vi "ATS_MS_Set_Device.vi"(8 "Update_Only":bool, 9 "Set_Manually (F)":bool, 10 "Setup_In":T1={"Record"={"Count"=1, "Presize"=512, "Length"=4096}, "Clock"={"ClckSource"=enum."Internal", "ClckRate"=12, "ClckEdge"=0, "Decimation"=0}, "Input A"={"Coupling"=enum."DC", "Range"=8, "Impedance"=enum."1M ohms", "Bandwidth"=enum."Full Bandwidth"}, "Input B"={"Coupling"=enum."DC", "Range"=8, "Impedance"=enum."1M ohms", "Bandwidth"=enum."Full Bandwidth"}, "Trigger"={"TrigOperation"=enum."X or Y", "Timeout (s)"=-1.0, "Trig. Delay"=0, "Engine X"={"Source"=enum."Chan_A", "Slope"=enum."Positive", "Level"=128}, "Engine Y"={"Source"=enum."Disable", "Slope"=enum."Positive", "Level"=128}, "ExtTrigControl"={"Coupling"=enum."AC", "Range"=enum."1 V"}}} {"Clock"."ClckEdge" items=["Rising", "Falling"]; "Clock"."ClckRate" items=["1 kS/s", "2 kS/s", "5 kS/s", "10 kS/s", "20 kS/s", "50 kS/s", "100 kS/s", "200 kS/s", "500 kS/s", "1 MS/s", "2 MS/s", "5 MS/s", "10 MS/s", "20 MS/s", "50 MS/s", "100 MS/s", "250 MS/s", "500 MS/s"]; "Input B"."Range" items=["40mV", "100mV", "200mV", "400mV", "1 V", "2 V", "4 V"]; "Trigger"."Timeout (s)" format="%.2f"; "Input A"."Range" items=["40mV", "100mV", "200mV", "400mV", "1 V", "2 V", "4 V"]}, 11 "DeviceIn":i32) -> (0 "error out":errorcluster={"status"=TRUE, "code"=60, "source"="ATS :     ApiInvalidHandle"}, 1 "Clock_Value (s)":dbl format="%.2p", 2 "Setup_Out":T1={"Record"={"Count"=1, "Presize"=512, "Length"=4096}, "Clock"={"ClckSource"=enum."Internal", "ClckRate"=12, "ClckEdge"=0, "Decimation"=0}, "Input A"={"Coupling"=enum."DC", "Range"=8, "Impedance"=enum."1M ohms", "Bandwidth"=enum."Full Bandwidth"}, "Input B"={"Coupling"=enum."DC", "Range"=8, "Impedance"=enum."1M ohms", "Bandwidth"=enum."Full Bandwidth"}, "Trigger"={"TrigOperation"=enum."X or Y", "Timeout (s)"=0.032768000000000005, "Trig. Delay"=0, "Engine X"={"Source"=enum."Chan_A", "Slope"=enum."Positive", "Level"=128}, "Engine Y"={"Source"=enum."Disable", "Slope"=enum."Positive", "Level"=128}, "ExtTrigControl"={"Coupling"=enum."AC", "Range"=enum."1 V"}}} {"Clock"."ClckEdge" items=["Rising", "Falling"]; "Clock"."ClckRate" items=["1 kS/s", "2 kS/s", "5 kS/s", "10 kS/s", "20 kS/s", "50 kS/s", "100 kS/s", "200 kS/s", "500 kS/s", "1 MS/s", "2 MS/s", "5 MS/s", "10 MS/s", "20 MS/s", "50 MS/s", "100 MS/s", "250 MS/s", "500 MS/s"]; "Input B"."Range" items=["20mv", "40mV", "50mV", "80mV", "100mV", "200mV", "400mV", "500mV", "800mV", "1 V", "2 V", "4 V", "5 V", "8 V", "10 V", "20 V"]; "Trigger"."Timeout (s)" max=0.0 format="%.2f"; "Input A"."Range" items=["20mv", "40mV", "50mV", "80mV", "100mV", "200mV", "400mV", "500mV", "800mV", "1 V", "2 V", "4 V", "5 V", "8 V", "10 V", "20 V"]}, 3 "DeviceOut":i32, 4 "TimeOut":dbl format="%.2f", 5 "#Device":i32)   [LabVIEW 2010]
doc: "_____AlazarTech, Scope_____\n\nSet ATS device with Setup_In parameters.\nIf Set_Manually is TRUE : Front panel open and the user can change setting.\nIf Set_Manually is FALSE: \n - update using input parameters.\n If UPDATE_Only is TRUE: update from previous set parameters"
uses:
  ATS_ctl/ATS_Global.ctl
  ATS_ctl/Record.ctl
  ATS_ctl/Clock.ctl
  ATS_ctl/ClockSource.ctl
  ATS_ctl/ClockRate.ctl
  ATS_ctl/ClockEdge.ctl
  ATS_ctl/InputCtrl.ctl
  ATS_ctl/Coupling.ctl
  ATS_ctl/Range.ctl
  ATS_ctl/Impedance.ctl
  ATS_ctl/Bandwidth.ctl
  ATS_ctl/Trigger.ctl
  ATS_ctl/TriggerOperation.ctl
  ATS_ctl/TriggerEngine.ctl
  ATS_ctl/ExtTrigger.ctl
  ATS_ctl/ExtTrigRange.ctl
  ATS_ctl/ATS_Spec_Selector.ctl
  ATS_ctl/ATS_Global_Ctrl.ctl
panel:
  out "Board":string
  out "Device":i32
  in  "String":string="Set parameters then push \"Continue ==>\""
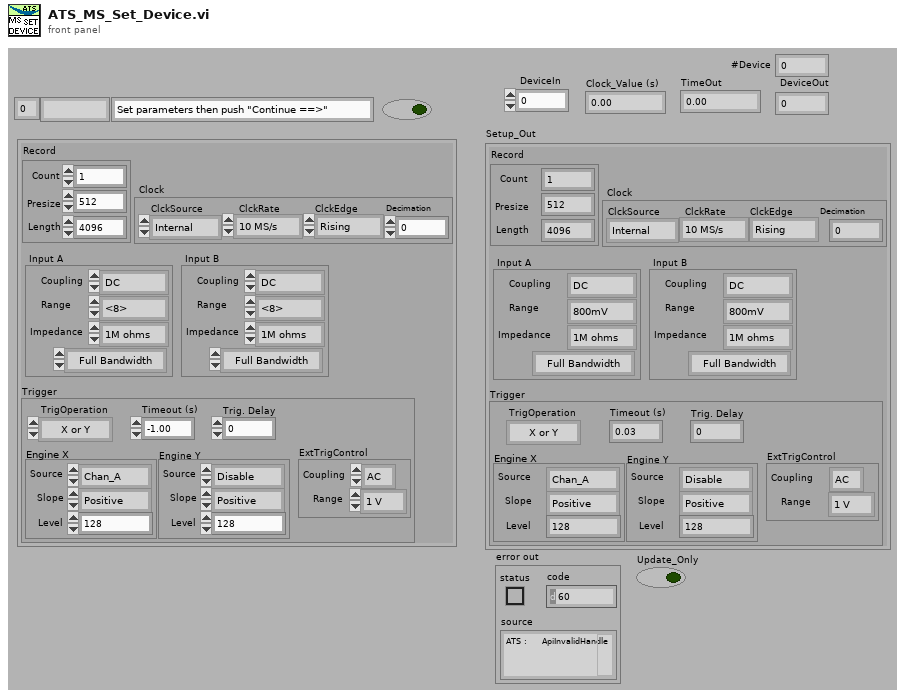
[diagram p1: front panel]
types:
  T1 = typedef "ATS_Global.ctl" = cluster{"Record":T2, "Clock":T3, "Input A":T7, "Input B":T7, "Trigger":T12}
  T2 = typedef "Record.ctl" = cluster{"Count":u32, "Presize":u32, "Length":u32}
  T3 = typedef "Clock.ctl" = cluster{"ClckSource":T4, "ClckRate":T5, "ClckEdge":T6, "Decimation":u32}
  T4 = typedef "ClockSource.ctl" = enum16{"Internal", "External", "Medium Ext.", "Slow Ext.", "Ext. AC", "Ext. DC", "Ext. (PLL)"}
  T5 = typedef "ClockRate.ctl" = u32
  T6 = typedef "ClockEdge.ctl" = u16
  T7 = typedef "InputCtrl.ctl" = cluster{"Coupling":T8, "Range":T9, "Impedance":T10, "Bandwidth":T11}
  T8 = typedef "Coupling.ctl" = enum16{"AC", "DC"}
  T9 = typedef "Range.ctl" = u32
  T10 = typedef "Impedance.ctl" = enum16{"1M ohms", "50 ohms"}
  T11 = typedef "Bandwidth.ctl" = enum16{"Full Bandwidth", "Reduce Bandwidth"}
  T12 = typedef "Trigger.ctl" = cluster{"TrigOperation":T13, "Timeout (s)":dbl, "Trig. Delay":u32, "Engine X":T14, "Engine Y":T14, "ExtTrigControl":T15}
  T13 = typedef "TriggerOperation.ctl" = enum16{"Only X", "Only Y", "X or Y", "X and Y", "X xor Y", "X and not Y", "not X and Y"}
  T14 = typedef "TriggerEngine.ctl" = cluster{"Source":enum32{"Chan_A", "Chan_B", "External", "Disable"}, "Slope":enum32{"Positive", "Negative"}, "Level":u32}
  T15 = typedef "ExtTrigger.ctl" = cluster{"Coupling":T8, "Range":T16}
  T16 = typedef "ExtTrigRange.ctl" = enum16{"1 V", "5 V", "TTL"}
  T17 = typedef "ATS_Spec_Selector.ctl" = enum16{"None", "ClckSource", "ClckEdge", "ClckRate", "InputRange", "InputCoupling", "Impedance", "Bandwidth", "AsyncDMA", "Memory", "ExtTrigCoupling", "ExtTrigRange", "AUX_IO_Trig", "AUX_IO_Slope", "Trigger_Source"}
  T18 = typedef "ATS_Global_Ctrl.ctl" = enum16{"Init_Device", "Clear_ALL", "Set", "Get"}
  T19 = typedef "ATS_Global_4Ch.ctl" = cluster{"Record":T2, "Clock":T3, "Inputs":T20, "Trigger":T21}
  T20 = typedef "ATS_InputArray.ctl" = T7[]
  T21 = typedef "ATS_Trigger_4Ch.ctl" = cluster{"TrigOperation":T13, "Timeout (s)":dbl, "Trig. Delay":u32, "Engine X":T22, "Engine Y":T22, "ExtTrigControl":T15}
  T22 = typedef "ATS_TriggerEngine_4Ch.ctl" = cluster{"Source":T23, "Slope":enum32{"Positive", "Negative"}, "Level":u32}
  T23 = typedef "ATS_TriggerSource_4Ch.ctl" = enum32{"Chan_A", "Chan_B", "External", "Disable", "Chan_C", "Chan_D"}
  T24 = cluster{"Record":T2, "Clock":T3, "OutputControl":T7, "OutputControl":T7, "Trigger":T21}
  T25 = typedef "Device_Info.ctl" = cluster{"Handle":u32, "Board":string, "CPLD":string, "MemorySize":u32, "SampleSize":u8, "ID":i32, "High_Memory":bool, "Chan/Board":u8}
  T26 = typedef "ATS_Sys_Info.ctl" = cluster{"MS_Mode":bool, "MBoard":i32, "#Board":i32}
  T27 = cluster{"Record":T2, "Clock":T3, "InputControl":T7, "InputControl":T7, "Trigger":T21}
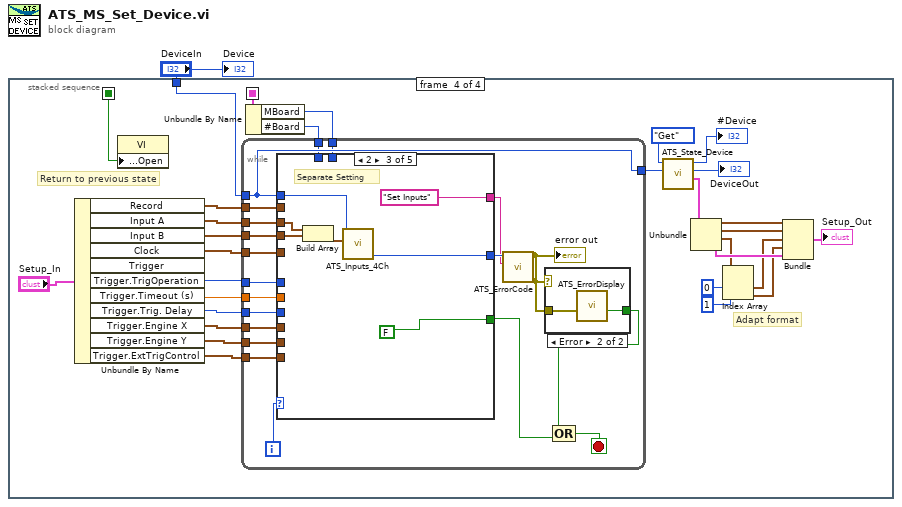
[diagram p0: block diagram]
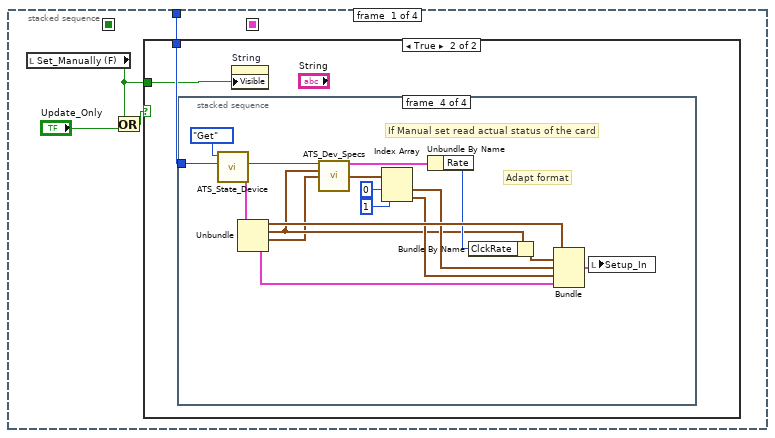
[diagram p2: hidden frame]
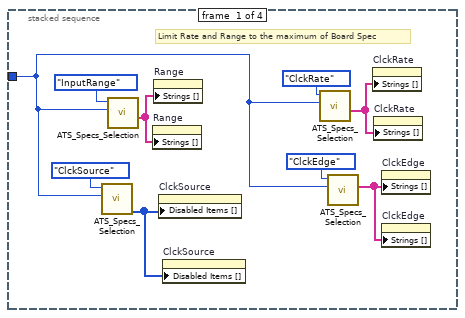
[diagram p4: hidden frame]
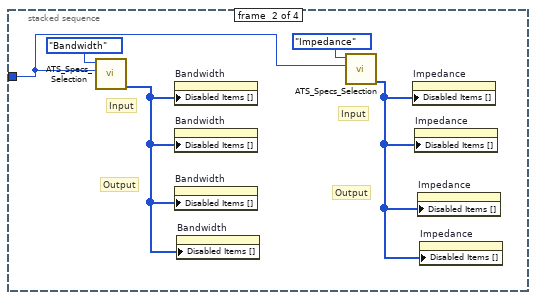
[diagram p5: hidden frame]
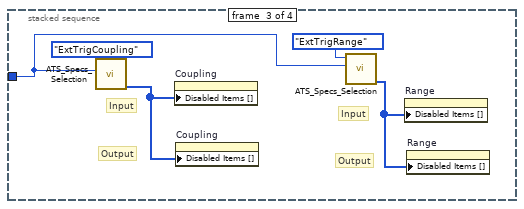
[diagram p6: hidden frame]
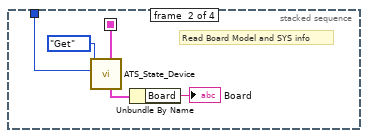
[diagram p7: hidden frame]
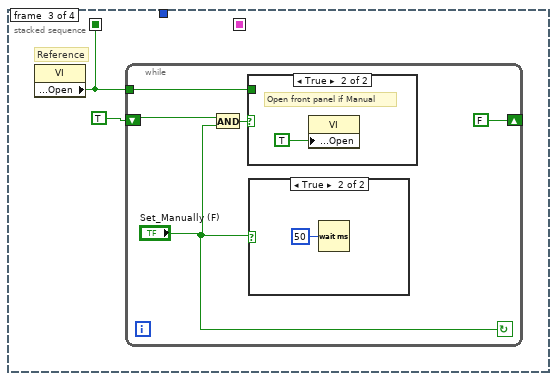
[diagram p8: hidden frame]
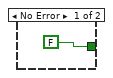
[diagram p11: hidden frame]
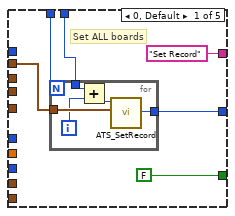
[diagram p12: hidden frame]
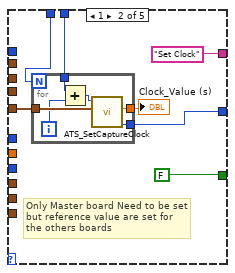
[diagram p13: hidden frame]
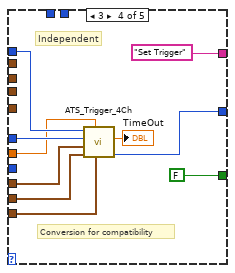
[diagram p14: hidden frame]
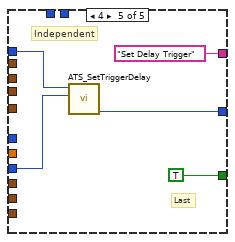
[diagram p15: hidden frame]
diagram:
  n1 = stacked-sequence {
    seq-local: [_ _ w49 _] -> [_ _ _ w76]
    seq-local: [_ w45 _ _] -> [_ _ _ w68]
    tunnel: "DeviceIn" -> [w5 w44 _ w71]
    frame #0 {
      n2 = local read "Set_Manually (F)"() -> (w2:bool)
      n3 = Or(x=w2, y="Update_Only") -> (x .or. y?=w4:bool)
      n4 = case shown="True" w4 {
        tunnel: w5 -> [_ w7]
        tunnel: w2 -> [_ w6]
        frame False {
        }
        frame True {
          n5 = stacked-sequence {
            tunnel: w7 -> [w10 w19 w22 w28]
            frame #0 {
              # "Limit Rate and Range to the maximum of Board Spec"
              n6 = call "ATS_Specs_Selection.vi"("Device"=w10, "ATS_Spec_Selector"=ATS_Spec_Selector."ClckSource") -> ("Disabled_Item"=w9:i32[])  [unwired: 3 in, 6 out]
              n7 = call "ATS_Specs_Selection.vi"("Device"=w10, "ATS_Spec_Selector"=ATS_Spec_Selector."InputRange") -> ("Possible_Item"=w16:string[])  [unwired: 3 in, 6 out]
              n8 = property on="Range" class="Ring (strict)"("Strings []"=w16) -> ()  [unwired: 2 in, 2 out]
              n9 = property on="Range" class="Ring (strict)"("Strings []"=w16) -> ()  [unwired: 2 in, 2 out]
              n10 = property on="ClckSource" class="Enum (strict)"("Disabled Items []"=w9) -> ()  [unwired: 2 in, 2 out]
              n11 = property on="ClckSource" class="Enum (strict)"("Disabled Items []"=w9) -> ()  [unwired: 2 in, 2 out]
              n12 = call "ATS_Specs_Selection.vi"("Device"=w10, "ATS_Spec_Selector"=ATS_Spec_Selector."ClckRate") -> ("Possible_Item"=w14:string[])  [unwired: 3 in, 6 out]
              n13 = call "ATS_Specs_Selection.vi"("Device"=w10, "ATS_Spec_Selector"=ATS_Spec_Selector."ClckEdge") -> ("All_Item"=w8:string[])  [unwired: 3 in, 6 out]
              n14 = property on="ClckRate" class="Ring (strict)"("Strings []"=w14) -> ()  [unwired: 2 in, 2 out]
              n15 = property on="ClckRate" class="Ring (strict)"("Strings []"=w14) -> ()  [unwired: 2 in, 2 out]
              n16 = property on="ClckEdge" class="Ring (strict)"("Strings []"=w8) -> ()  [unwired: 2 in, 2 out]
              n17 = property on="ClckEdge" class="Ring (strict)"("Strings []"=w8) -> ()  [unwired: 2 in, 2 out]
            }
            frame #1 {
              # "Output"
              # "Input"
              # "Output"
              # "Input"
              n18 = call "ATS_Specs_Selection.vi"("Device"=w19, "ATS_Spec_Selector"=ATS_Spec_Selector."Bandwidth") -> ("Disabled_Item"=w18:i32[])  [unwired: 3 in, 6 out]
              n19 = property on="Bandwidth" class="Enum (strict)"("Disabled Items []"=w18) -> ()  [unwired: 2 in, 2 out]
              n20 = property on="Bandwidth" class="Enum (strict)"("Disabled Items []"=w18) -> ()  [unwired: 2 in, 2 out]
              n21 = property on="Bandwidth" class="Enum (strict)"("Disabled Items []"=w18) -> ()  [unwired: 2 in, 2 out]
              n22 = property on="Bandwidth" class="Enum (strict)"("Disabled Items []"=w18) -> ()  [unwired: 2 in, 2 out]
              n23 = call "ATS_Specs_Selection.vi"("Device"=w19, "ATS_Spec_Selector"=ATS_Spec_Selector."Impedance") -> ("Disabled_Item"=w17:i32[])  [unwired: 3 in, 6 out]
              n24 = property on="Impedance" class="Enum (strict)"("Disabled Items []"=w17) -> ()  [unwired: 2 in, 2 out]
              n25 = property on="Impedance" class="Enum (strict)"("Disabled Items []"=w17) -> ()  [unwired: 2 in, 2 out]
              n26 = property on="Impedance" class="Enum (strict)"("Disabled Items []"=w17) -> ()  [unwired: 2 in, 2 out]
              n27 = property on="Impedance" class="Enum (strict)"("Disabled Items []"=w17) -> ()  [unwired: 2 in, 2 out]
            }
            frame #2 {
              # "Output"
              # "Input"
              # "Output"
              # "Input"
              n28 = call "ATS_Specs_Selection.vi"("Device"=w22, "ATS_Spec_Selector"=ATS_Spec_Selector."ExtTrigCoupling") -> ("Disabled_Item"=w24:i32[])  [unwired: 3 in, 6 out]
              n29 = property on="Coupling" class="Enum (strict)"("Disabled Items []"=w24) -> ()  [unwired: 2 in, 2 out]
              n30 = property on="Coupling" class="Enum (strict)"("Disabled Items []"=w24) -> ()  [unwired: 2 in, 2 out]
              n31 = call "ATS_Specs_Selection.vi"("Device"=w22, "ATS_Spec_Selector"=ATS_Spec_Selector."ExtTrigRange") -> ("Disabled_Item"=w23:i32[])  [unwired: 3 in, 6 out]
              n32 = property on="Range" class="Enum (strict)"("Disabled Items []"=w23) -> ()  [unwired: 2 in, 2 out]
              n33 = property on="Range" class="Enum (strict)"("Disabled Items []"=w23) -> ()  [unwired: 2 in, 2 out]
            }
            frame #3 {
              # "Adapt format"
              # "If Manual set read actual status of the card"
              n34 = call "ATS_State_Device.vi"("DeviceIn"=w28, "ATS_GBL_Ctrl"=ATS_Global_Ctrl."Get") -> ("SetupOut"=w37:T19, "DeviceOut"=w27:i32)  [unwired: 4 in, 4 out]
              n35 = Unbundle(w37) -> ("Record"=w36:T2, "Clock"=w30:T3, "Inputs"=w29:T20, "Trigger"=w31:T21)
              n36 = call "ATS_Dev_Specs.vi"("Device"=w27, "Clock"=w30, "Input_Chan"=w29) -> ("Rate_Out"=w42:cluster{"Text":string, "Rate":i32}, "Output_Chan"=w41:T7[])  [unwired: 8 in, 3 out]
              n37 = Index Array(array=w41, index #1=0 ("index"), index #2=1 ("index")) -> (element #1=w33:T7, element #2=w32:T7)
              n38 = Unbundle By Name(w42) -> ("Rate"=w35:i32)
              n39 = Bundle By Name(cluster=w30, "ClckRate"=w35) -> (w34:T3)
              n40 = Bundle("Record"=w36, "Clock"=w34, "OutputControl"=w33, "OutputControl"=w32, "Trigger"=w31) -> (w38:T24)  [unwired: 1 in]
              n41 = local write "Setup_In"(w38) -> ()
            }
          }
          n42 = property on="String" class="Str"("Visible"=w6) -> ()  [unwired: 2 in, 2 out]
        }
      }
    }
    frame #1 {
      # "Read Board Model and SYS info"
      n43 = call "ATS_State_Device.vi"("DeviceIn"=w44, "ATS_GBL_Ctrl"=ATS_Global_Ctrl."Get") -> ("DevInfo_Out"=w48:T25, "Sys_Out"=w45:T26)  [unwired: 4 in, 4 out]
      n44 = Unbundle By Name(w48) -> ("Board"=→"Board":string)
    }
    frame #2 {
      # "Reference"
      n45 = property class="VI"() -> ("Front Panel Window:Open"=w49:bool)  [unwired: 2 in, 2 out]
      n46 = while {
        shift-right: [FALSE ("Front Panel Window:Open")] -> _
        shift-left: TRUE ("Front Panel Window:Open") -> [w54]
        tunnel: w49 -> [w53]
        stop <- "Set_Manually (F)" continue-if-true
        n47 = And(x=w54, y="Set_Manually (F)") -> (x .and. y?=w52:bool)
        n48 = case shown="True" w52 {
          tunnel: w53 -> [_ _]
          frame False {
          }
          frame True {
            # "Open front panel if Manual"
            n49 = property class="VI"("Front Panel Window:Open"=TRUE) -> ()  [unwired: 2 in, 2 out]
          }
        }
        n50 = case shown="True" "Set_Manually (F)" {
          frame False {
            # "No Stop"
          }
          frame True {
            n51 = Wait (ms)(milliseconds to wait=u32 50) -> ()  [unwired: 1 out]
          }
        }
      }
    }
    frame #3 {
      # "Adapt format"
      # "Return to previous state"
      n52 = Unbundle By Name("Setup_In") -> ("Record"=w86:T2, "Input A"=w84:T7, "Input B"=w83:T7, "Clock"=w85:T3, "Trigger.TrigOperation"=w79:T13, "Trigger.Timeout (s)"=w78:dbl, "Trigger.Trig. Delay"=w77:u32, "Trigger.Engine X"=w80:T14, "Trigger.Engine Y"=w81:T14, "Trigger.ExtTrigControl"=w82:T15)  [unwired: 1 out]
      n53 = property class="VI"("Front Panel Window:Open"=w76) -> ()  [unwired: 2 in, 2 out]
      n54 = Unbundle By Name(w68) -> ("MBoard"=w70:i32, "#Board"=w69:i32)
      n55 = while {
        tunnel: w71 -> [w94]
        tunnel: w86 -> [w104]
        tunnel: w85 -> [w103]
        tunnel: w84 -> [w102]
        tunnel: w83 -> [w101]
        tunnel: w82 -> [w100]
        tunnel: w81 -> [w99]
        tunnel: w80 -> [w98]
        tunnel: w79 -> [w97]
        tunnel: w78 -> [w96]
        tunnel: w77 -> [w95]
        tunnel: [w94] -> w75
        tunnel: w70 -> [w89]
        tunnel: w69 -> [w88]
        i -> [w90]
        stop <- w93 stop-if-true
        n56 = case shown="2" w90 {
          tunnel: [w116 w128 w140 w149 w156] -> w107
          tunnel: w94 -> [_ _ w141 w150 w154]
          tunnel: [FALSE ("value") FALSE ("value") FALSE ("value") FALSE ("value") TRUE ("value")] -> w92
          tunnel: w104 -> [w114 _ _ _ _]
          tunnel: w103 -> [_ w126 _ _ _]
          tunnel: w102 -> [_ _ w136 _ _]
          tunnel: w101 -> [_ _ w135 _ _]
          tunnel: w100 -> [_ _ _ w148 _]
          tunnel: w99 -> [_ _ _ w147 _]
          tunnel: w98 -> [_ _ _ w146 _]
          tunnel: w97 -> [_ _ _ w145 _]
          tunnel: w96 -> [_ _ _ w144 _]
          tunnel: w95 -> [_ _ _ _ w153]
          tunnel: ["Set Record" "Set Clock" "Set Inputs" "Set Trigger" "Set Delay Trigger"] -> w91
          tunnel: w89 -> [w112 w123 _ _ _]
          tunnel: w88 -> [w111 w122 _ _ _]
          frame 0, Default {
            # "Set ALL boards"
            n57 = for {
              N: w111 -> [_]
              tunnel: [w121] -> w116
              tunnel: w114 -> [w120]
              tunnel: w112 -> [w117]
              i -> [w118]
              n58 = Add(x=w117, y=w118) -> (x+y=w119:i32)
              n59 = call "ATS_SetRecord.vi"("RecordIn"=w120, "DeviceIn"=w119) -> ("Return Code"=w121:u32)  [unwired: 7 in, 2 out]
            }
          }
          frame 1 {
            # "Only Master board Need to be set\nbut reference value are set for\nthe others boards"
            n60 = for {
              N: w122 -> [_]
              tunnel: [w134] -> w128
              tunnel: w126 -> [w133]
              tunnel: [w132] -> w125
              tunnel: w123 -> [w129]
              i -> [w131]
              n61 = Add(x=w129, y=w131) -> (x+y=w130:i32)
              n62 = call "ATS_SetCaptureClock.vi"("Clock"=w133, "DeviceIn"=w130) -> ("Return Code"=w134:u32, "Clock_Value (s)"=w132:dbl)  [unwired: 7 in, 1 out]
            }
            "Clock_Value (s)" <- w125
          }
          frame 2 {
            # "Separate Setting"
            n63 = Build Array(w136, w135) -> (w137:T7[])
            n64 = call "ATS_Inputs_4Ch.vi"("Channels_Input"=w137, "DeviceIn"=w141) -> ("Return Code"=w140:u32)  [unwired: 5 in, 4 out]
          }
          frame 3 {
            # "Conversion for compatibility"
            # "Independent"
            n65 = call "ATS_Trigger_4Ch.vi"("ExtTrigControl"=w148, "Timeout (-1, Auto)"=w144, "Engine Y"=w147, "Engine X"=w146, "TrigOperation"=w145, "DeviceIn"=w150) -> ("Return Code"=w149:u32, "Timeout"=→"TimeOut":dbl)  [unwired: 3 in, 1 out]
          }
          frame 4 {
            # "Last"
            # "Independent"
            n66 = call "ATS_SetTriggerDelay.vi"("Delay"=w153, "DeviceIn"=w154) -> ("Return Code"=w156:u32)  [unwired: 8 in, 1 out]
          }
        }
        n67 = call "ATS_ErrorCode.vi"("Message"=w91, "ErrorCode"=w107) -> ("error out"=w105:errorcluster)  [unwired: 5 in]
        "error out" <- w105
        n68 = case shown="Error" w105 {
          tunnel: [FALSE ("End 2") w110] -> w106
          tunnel: w105 -> [_ w109]
          frame No Error {
          }
          frame Error {
            n69 = call "ATS_ErrorDisplay.vi"("error IN"=w109) -> ("End Out"=w110:bool)  [unwired: 6 in]
          }
        }
        n70 = Compound Arithmetic op=OR(w106, w92) -> (w93:bool)
      }
      n71 = call "ATS_State_Device.vi"("DeviceIn"=w75, "ATS_GBL_Ctrl"=ATS_Global_Ctrl."Get") -> ("SetupOut"=w66:T19, "DeviceOut"=→"DeviceOut":i32, "#Device"=→"#Device":i32)  [unwired: 4 in, 3 out]
      n72 = Unbundle(w66) -> ("Record"=w65:T2, "Clock"=w64:T3, "Inputs"=w60:T20, "Trigger"=w63:T21)
      n73 = Index Array(array=w60, index #1=0 ("index"), index #2=1 ("index")) -> (element #1=w59:T7, element #2=w58:T7)
      n74 = Bundle("Record"=w65, "Clock"=w64, "InputControl"=w59, "InputControl"=w58, "Trigger"=w63) -> (→"Setup_Out":T27)  [unwired: 1 in]
    }
  }
  "Device" <- "DeviceIn"
